vi "Process Control.vi"(5 "State in":T1, 6 "Name in":string, 7 "Action in":T2, 11 "Game Board in":refnum<class "Game Board.lvclass">) -> (3 "Game Board out":refnum<class "Game Board.lvclass">)   [LabVIEW 2024, in "Game Board.lvclass"]
doc: "MIT Licence\nCopyright (c) 2024 David Grollier"
uses:
  Game Board.lvclass
  Action Command.ctl
  State Command.ctl
  Game Board.lvclass/Game Board.ctl
  Game Board Component/Movable/Flying Saucer/Flying Saucer.lvclass
  Game Board Component/Movable/Flying Saucer/Flying Saucer.lvclass/Flying Saucer.ctl
  Game Board Component/Game Board Component.lvclass
  Game Board Component/Movable/Movable.lvclass
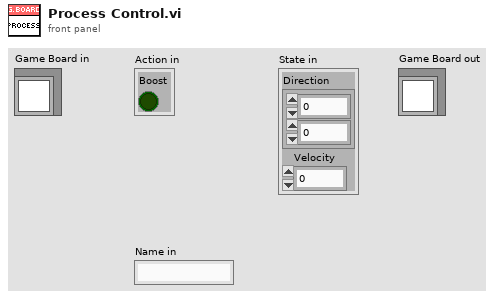
[diagram p1: front panel]
types:
  T1 = typedef "Game Board.lvclass/State Command.ctl" = cluster{"Direction":cluster{dbl, dbl}, "Velocity":dbl}
  T2 = typedef "Game Board.lvclass/Action Command.ctl" = cluster{"Boost":bool}
  T3 = map{string, refnum<class "Game Board Component.lvclass">}
  T4 = typedef "Velocity.ctl" = cluster{"Vx":dbl, "Vy":dbl}
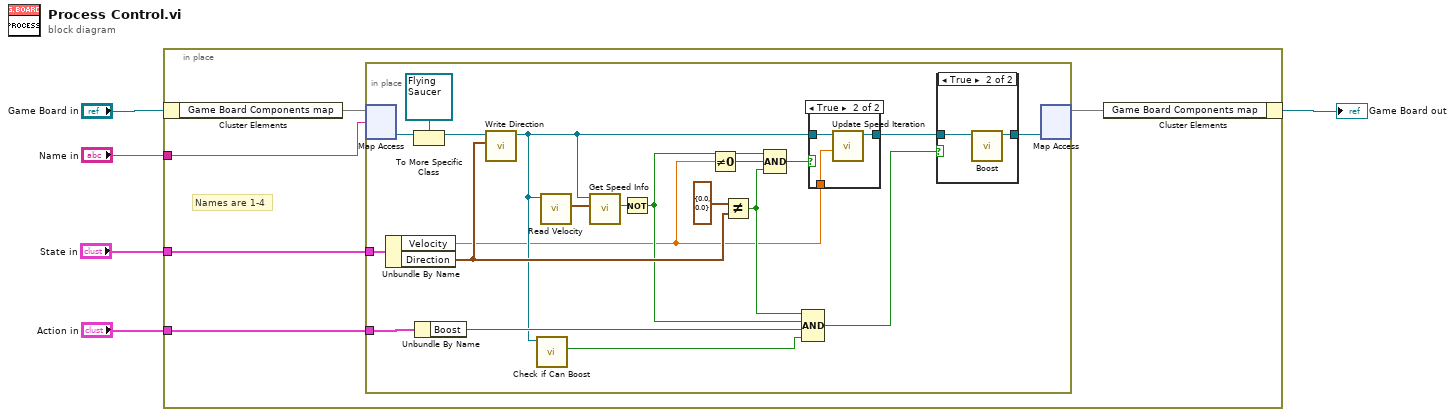
[diagram p0: block diagram]
diagram:
  n1 = in-place {
    in-place-border: "State in" -> [w9]
    in-place-border: "Action in" -> [w7]
    in-place-border: "Name in" -> [w6]
    # "Names are 1-4"
    n2 = in-place-cluster #1("Game Board in") -> ("Game Board Components map"=w10:T3)
    n3 = in-place {
      in-place-border: w9 -> [w28]
      in-place-border: w7 -> [w22]
      n4 = in-place-map #2(w10, w6) -> (w29:refnum<class "Game Board Component.lvclass">)  [unwired: 1 in, 1 out]
      n5 = Unbundle By Name(w28) -> ("Velocity"=w11:dbl, "Direction"=w18:cluster{dbl, dbl})
      n6 = To More Specific Class(target class=refnum<class "Flying Saucer.lvclass"> refnum ("Flying Saucer.lvclass"), reference=w29) -> (specific class reference=w27:refnum<class "Flying Saucer.lvclass">)  [unwired: 1 in, 1 out]
      n7 = Unbundle By Name(w22) -> ("Boost"=w21:bool)
      n8 = call "Write Direction.vi"("Velocity"=w18, "Flying Saucer in"=w27) -> ("Flying Saucer out"=w14:refnum<class "Flying Saucer.lvclass">)  [unwired: 9 in]
      n9 = call "Check if Can Boost.vi"("Flying Saucer in"=w14) -> ("Can Boost?"=w13:bool)  [unwired: 10 in]
      n10 = call-dynamic "Read Velocity.vi"("Movable in"=w14) -> ("Velocity"=w17:T4)  [unwired: 10 in]
      n11 = call "Get Speed Info.vi"("Velocity in"=w17, "Movable in"=w14) -> ("Max speed?"=w16:bool)  [unwired: 8 in, 1 out]
      n12 = Not(x=w16) -> (.not. x?=w15:bool)
      n13 = Not Equal To 0?(x=w11) -> (x != 0?=w20:bool)
      n14 = Not Equal?(x=cluster{dbl, dbl} {0.0, 0.0}, y=w18) -> (x != y?=w19:bool)
      n15 = Compound Arithmetic op=AND(w15, w20, w19) -> (w25:bool)
      n16 = Compound Arithmetic op=AND(w19, w15, w21, w13) -> (w12:bool)
      n17 = case shown="True" w25 {
        tunnel: w14 -> [w31 w34]
        tunnel: [w31 w33] -> w24
        tunnel: w11 -> [_ w32]
        frame False {
        }
        frame True {
          n18 = call "Update Speed Iteration.vi"("Triggers in"=w32, "Flying Saucer in"=w34) -> ("Flying Saucer out"=w33:refnum<class "Flying Saucer.lvclass">)  [unwired: 9 in]
        }
      }
      n19 = case shown="True" w12 {
        tunnel: w24 -> [w35 w36]
        tunnel: [w35 w37] -> w23
        frame False {
        }
        frame True {
          n20 = call "Boost.vi"("Flying Saucer in"=w36) -> ("Flying Saucer out"=w37:refnum<class "Flying Saucer.lvclass">)  [unwired: 10 in]
        }
      }
      n21 = in-place-map #2(w23) -> (w8:T3)  [unwired: 1 in, 2 out]
    }
    n22 = in-place-cluster #1("Game Board Components map"=w8) -> (→"Game Board out":refnum<class "Game Board.lvclass">)
  }
